vi "test_Decode Raw Payload.vi"() -> ()   [LabVIEW 2020]
uses:
  <instrlib>/AIM GmbH/_AIM 664/_controls/queue_data_full.ctl
  <instrlib>/AIM GmbH/_AIM 664/AIM664LV.lvlib
panel:
  out "Frame Configuration":T1={"domainID"=1, "sideID"=1, "locationID"=1, "interfaceID"=1, "partitionID"=1} {"interfaceID" format="%.0b"}
  out "Payload":u8[](array[numeric])
  out "VL Id":u16=60
  out "UDPdstPort":u16=1
  out "UDPsrcPort":u16=1
  in  "Data":u8[](array[numeric])=[3, 0, 0, 0, 0, 60, 2, 0, 0, 1, 33, 32, 8, 0, 69, 0, 0, 60, 0, 0, 64, 0, 1, 17, 109, 147, 10, 1, 33, 1, 224, 224, 0, 60, 0, 23, 0, 24, 0, 40, 0, 0, 0, 0, 0, 0, 0, 0, 0, 0, 0, 0, 0, 0, 0, 0, 0, 0, 0, 0, 0, 0, 0, 0, 0, 0, 0, 0, 0, 0, 0, 0, 0, 0, 0, 0, 0, 0, 0] format="%.0x"
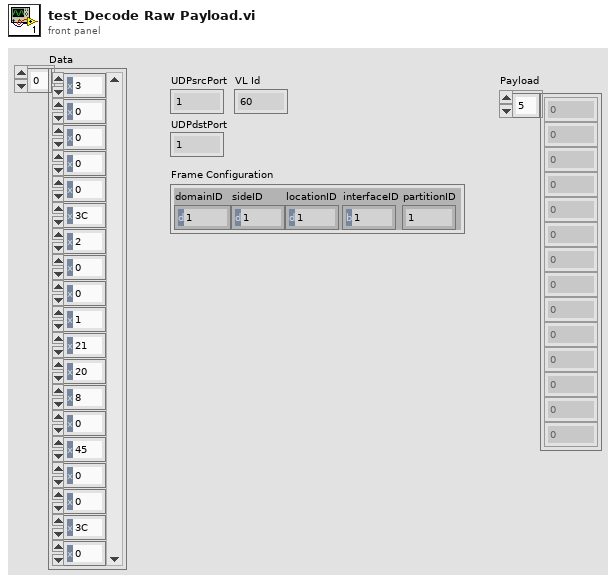
[diagram p1: front panel]
types:
  T1 = typedef "AIM664LV.lvlib/queue_data_full.ctl" = cluster{"domainID":u8, "sideID":u8, "locationID":u8, "interfaceID":u8, "partitionID":u8}
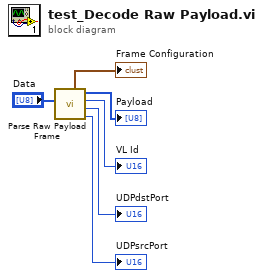
[diagram p0: block diagram]
diagram:
  n1 = call "Parse Raw Payload Frame.vi"("Data"="Data") -> ("UDPsrcPort"=→"UDPsrcPort":u16, "UDPdstPort"=→"UDPdstPort":u16, "VL Id"=→"VL Id":u16, "Payload"=→"Payload":u8[], "Frame Configuration"=→"Frame Configuration":T1)  [unwired: 6 in]
